vi "GetSlitwidth.vi"(8 "error in (no error)":errorcluster, 10 "Slit":T1(ring), 11 "HRS_Spectrometer in":refnum<class "HRS_Spectrometer.lvclass">) -> (0 "error out":errorcluster, 3 "HRS_Spectrometer out":refnum<class "HRS_Spectrometer.lvclass">)   [LabVIEW 2023, in "Spectrometer Library.lvlib" / "HRS_Spectrometer.lvlib" / "HRS_Spectrometer.lvclass"]
uses:
  HRS_Spectrometer.lvclass
  HRS_Spectrometer.lvclass/HRS_Spectrometer.ctl
  <vilib>/addons/Tools/Unicode/UTF8 Tools.lvlib
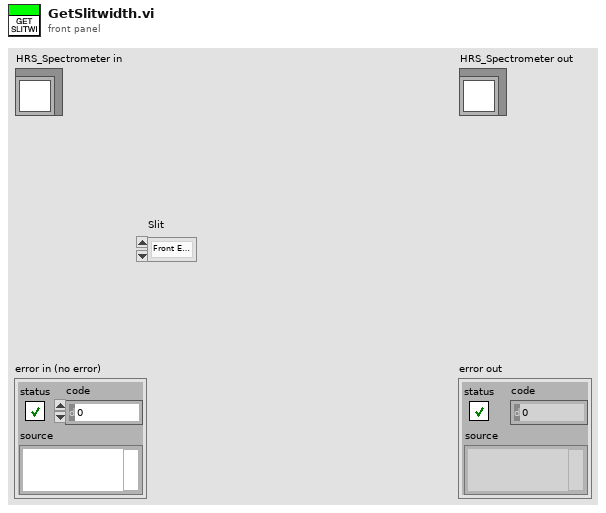
[diagram p1: front panel]
types:
  T1 = enum16{"Front Entrance Slit", "Side Entrance Slit", "Front Exit Slit", "Side Exit Slit"}
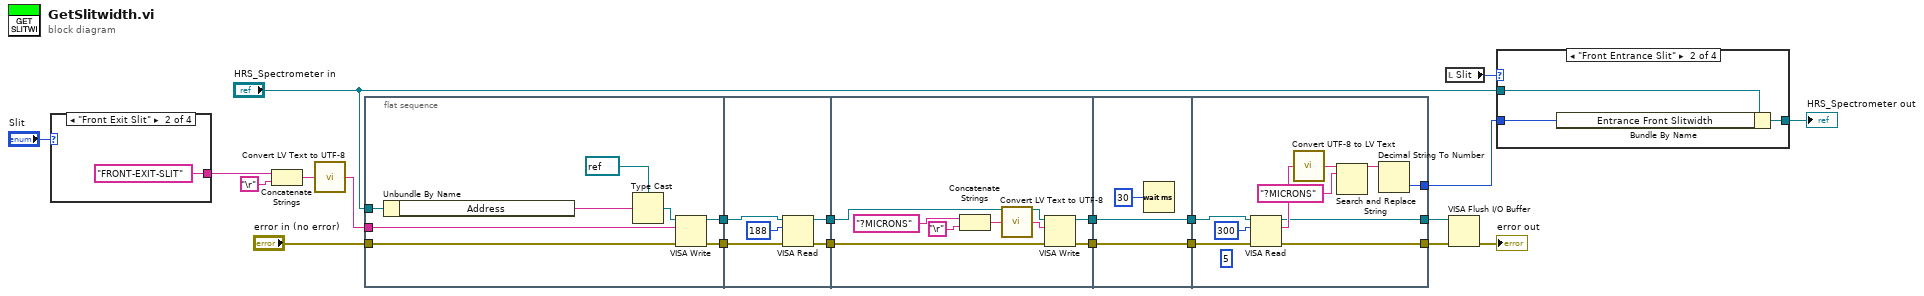
[diagram p0: block diagram]
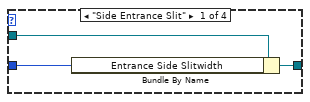
[diagram p2: hidden frame]
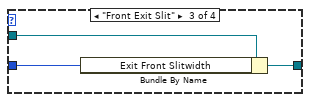
[diagram p3: hidden frame]
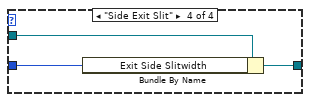
[diagram p4: hidden frame]
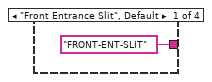
[diagram p5: hidden frame]
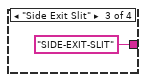
[diagram p6: hidden frame]
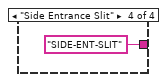
[diagram p7: hidden frame]
diagram:
  n1 = case shown="\"Front Exit Slit\"" "Slit" {
    tunnel: ["FRONT-ENT-SLIT" "FRONT-EXIT-SLIT" "SIDE-EXIT-SLIT" "SIDE-ENT-SLIT"] -> w6
    frame "Front Entrance Slit", Default {
    }
    frame "Front Exit Slit" {
    }
    frame "Side Exit Slit" {
    }
    frame "Side Entrance Slit" {
    }
  }
  n2 = Concatenate Strings(w6, "\r") -> (w4:string)
  n3 = call <vilib>:"Convert LV Text to UTF-8.vi"("LV Text"=w4) -> ("UTF-8 Text"=w7:string)  [unwired: 13 in, 1 out]
  n4 = flat-sequence {
    tunnel: "HRS_Spectrometer in" -> [w33]
    tunnel: w7 -> [w32]
    tunnel: [w31] -> w20
    tunnel: [w30] -> w19
    tunnel: "error in (no error)" -> [w29]
    tunnel: w20 -> [w38]
    tunnel: w19 -> [w37]
    tunnel: [w36] -> w18
    tunnel: [w35] -> w17
    tunnel: w18 -> [w45]
    tunnel: w17 -> [w46]
    tunnel: [w44] -> w11
    tunnel: [w43] -> w8
    tunnel: w11 -> [w48]
    tunnel: [w48] -> w10
    tunnel: [w47] -> w9
    tunnel: w8 -> [w47]
    tunnel: [w58] -> w12
    tunnel: w10 -> [w57]
    tunnel: w9 -> [w56]
    tunnel: [w54] -> w3
    tunnel: [w50] -> w1
    frame #0 {
      n5 = Unbundle By Name(w33) -> ("Address"=w27:string)
      n6 = Type Cast(type=refnum<visa-resource-name> refnum ("VISA resource name out"), x=w27) -> (*(type *) &x=w26:refnum<visa-resource-name>)
      n7 = VISA Write(VISA resource name=w26, write buffer=w32, error in (no error)=w29) -> (VISA resource name out=w31:refnum<visa-resource-name>, error out=w30:errorcluster)  [unwired: 1 out]
    }
    frame #1 {
      n8 = VISA Read(VISA resource name=w38, byte count=u32 188, error in (no error)=w37) -> (VISA resource name out=w36:refnum<visa-resource-name>, error out=w35:errorcluster)  [unwired: 2 out]
    }
    frame #2 {
      n9 = Concatenate Strings("?MICRONS" ("write buffer"), "\r") -> (w39:string)
      n10 = call <vilib>:"Convert LV Text to UTF-8.vi"("LV Text"=w39) -> ("UTF-8 Text"=w42:string)  [unwired: 13 in, 1 out]
      n11 = VISA Write(VISA resource name=w45, write buffer=w42, error in (no error)=w46) -> (VISA resource name out=w43:refnum<visa-resource-name>, error out=w44:errorcluster)  [unwired: 1 out]
    }
    frame #3 {
      n12 = Wait (ms)(milliseconds to wait=u32 30) -> ()  [unwired: 1 out]
    }
    frame #4 {
      (unwired) u32 5 ("byte count")
      n13 = VISA Read(VISA resource name=w56, byte count=u32 300, error in (no error)=w57) -> (VISA resource name out=w54:refnum<visa-resource-name>, read buffer=w55:string, error out=w50:errorcluster)  [unwired: 1 out]
      n14 = call <vilib>:"Convert UTF-8 to LV Text.vi"("UTF-8 Text"=w55) -> ("LV Text"=w53:string)  [unwired: 13 in, 1 out]
      n15 = Search and Replace String(input string=w53, search string="?MICRONS" ("write buffer")) -> (result string=w51:string)  [unwired: 6 in, 3 out]
      n16 = Decimal String To Number(string=w51) -> (number=w58:i32)  [unwired: 2 in, 1 out]
    }
  }
  n17 = local read "Slit"() -> (w15:T1)
  n18 = VISA Flush I/O Buffer(VISA resource name=w3, error in (no error)=w1) -> (error out=→"error out":errorcluster)  [unwired: 1 in, 1 out]
  n19 = case shown="\"Front Entrance Slit\"" w15 {
    tunnel: "HRS_Spectrometer in" -> [w62 w65 w68 w71]
    tunnel: w12 -> [w61 w64 w67 w70]
    tunnel: [w60 w63 w66 w69] -> w14
    frame "Side Entrance Slit" {
      n20 = Bundle By Name(cluster=w62, "Entrance Side Slitwidth"=w61) -> (w60:refnum<class "HRS_Spectrometer.lvclass">)
    }
    frame "Front Entrance Slit" {
      n21 = Bundle By Name(cluster=w65, "Entrance Front Slitwidth"=w64) -> (w63:refnum<class "HRS_Spectrometer.lvclass">)
    }
    frame "Front Exit Slit" {
      n22 = Bundle By Name(cluster=w68, "Exit Front Slitwidth"=w67) -> (w66:refnum<class "HRS_Spectrometer.lvclass">)
    }
    frame "Side Exit Slit" {
      n23 = Bundle By Name(cluster=w71, "Exit Side Slitwidth"=w70) -> (w69:refnum<class "HRS_Spectrometer.lvclass">)
    }
  }
  "HRS_Spectrometer out" <- w14
